vi "Untitled 1.vi"() -> ()   [LabVIEW 2012]
panel:
  out "gravity":string
  out "work of compressor":dbl
  out "density":dbl
  out "pressure":dbl(knob) scale=0.0..1.0
  out "temp":dbl(knob) scale=-40.0..-30.0
  in  "height":dbl
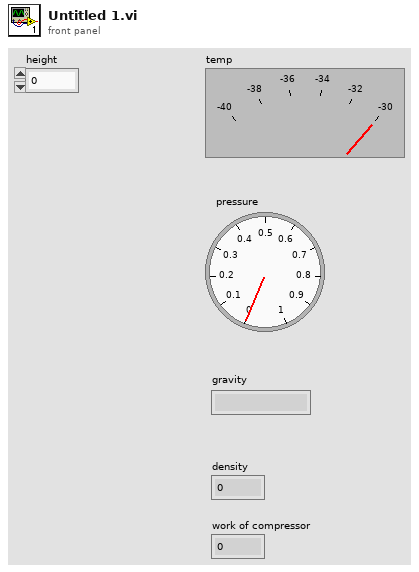
[diagram p1: front panel]
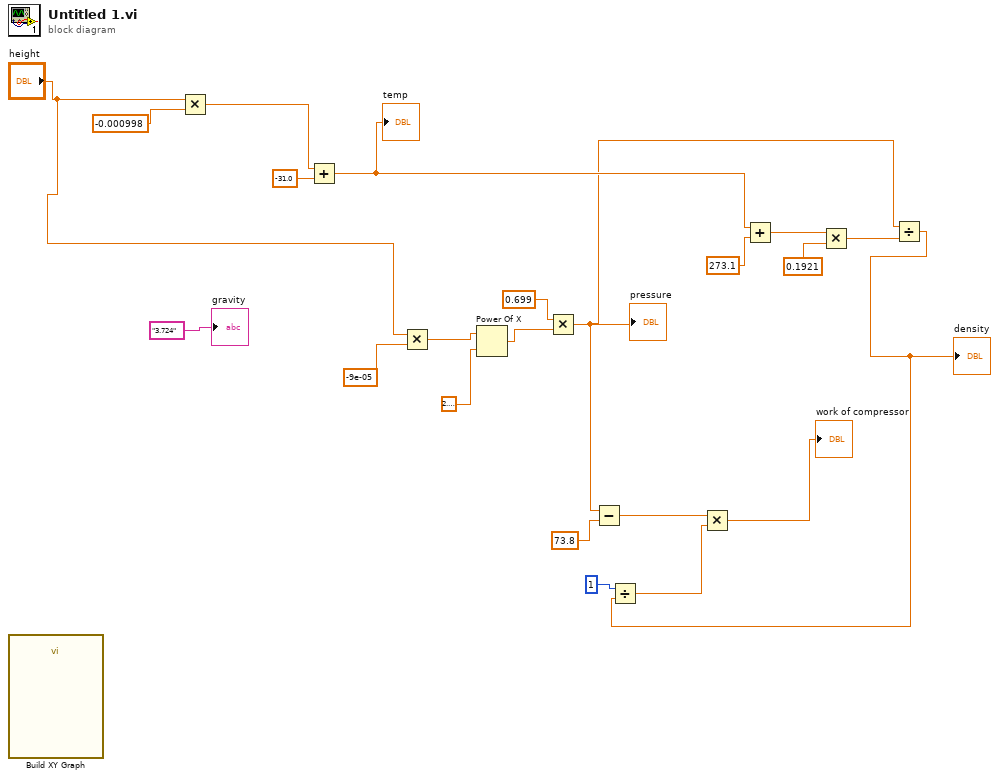
[diagram p0: block diagram]
diagram:
  n1 = call "Build XY Graph"() -> ("XY Graph"=w1:cluster{"Y":dbl[], "Y":dbl[]}[])  [unwired: 5 in, 6 out]
  n2 = Multiply(x="height", y=-0.000998) -> (x*y=w22:dbl)
  n3 = Add(x=w22, y=-31.0) -> (x+y=w13:dbl)
  "temp" <- w13
  n4 = Multiply(x="height", y=-9e-05) -> (x*y=w18:dbl)
  n5 = Power Of X(1:2.718281828459045, 2:w18) -> (0:w16:dbl)
  n6 = Multiply(x=0.699, y=w16) -> (x*y=w8:dbl)
  "pressure" <- w8
  n7 = Subtract(x=w8, y=73.8) -> (x-y=w7:dbl)
  n8 = Add(x=w13, y=273.1) -> (x+y=w12:dbl)
  n9 = Multiply(x=w12, y=0.1921) -> (x*y=w10:dbl)
  n10 = Divide(x=w8, y=w10) -> (x/y=w6:dbl)
  "density" <- w6
  n11 = Divide(x=1, y=w6) -> (x/y=w4:dbl)
  n12 = Multiply(x=w7, y=w4) -> (x*y=→"work of compressor":dbl)
  "gravity" <- "3.724"
